vi "test_libssh2_session_blocking.vi"() -> ()   [LabVIEW 2013, in "libssh2_tests.lvlib"]
uses:
  libssh2/libssh2_init_default.vi
  libssh2_tests.lvlib
  <vilib>/addons/_JKI Toolkits/Caraya/classes/Test/Test.lvclass
  libssh2/libssh2.lvlib
  <vilib>/addons/_JKI Toolkits/Caraya/classes/Assert/Assert.lvclass
panel:
  out "error out":errorcluster
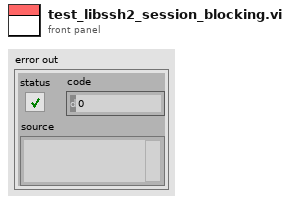
[diagram p1: front panel]
types:
  T1 = typedef "libssh2.lvlib/Session Refnum.ctl" = refnum<k1>
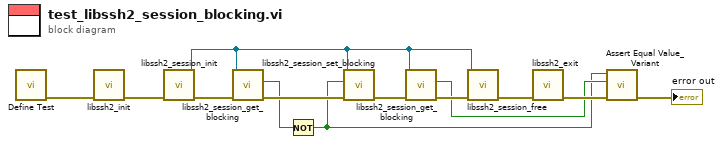
[diagram p0: block diagram]
diagram:
  n1 = call <vilib>:"Define Test.vi"() -> ("error out"=w8:errorcluster)  [unwired: 10 in, 1 out]
  n2 = call-poly "libssh2_init.vi"("error in (no error)"=w8) -> ("error out"=w12:errorcluster)  [unwired: 10 in]
  n3 = call "libssh2_session_init.vi"("error in (no error)"=w12) -> ("error out"=w5:errorcluster, "session"=w4:T1)  [unwired: 9 in]
  n4 = call "libssh2_session_get_blocking.vi"("error in (no error)"=w5, "session"=w4) -> ("error out"=w6:errorcluster, "blocking"=w3:bool)  [unwired: 8 in]
  n5 = Not(x=w3) -> (.not. x?=w1:bool)
  n6 = call "libssh2_session_set_blocking.vi"("error in (no error)"=w6, "blocking"=w1, "session"=w4) -> ("error out"=w10:errorcluster)  [unwired: 8 in]
  n7 = call "libssh2_session_get_blocking.vi"("error in (no error)"=w10, "session"=w4) -> ("error out"=w7:errorcluster, "blocking"=w2:bool)  [unwired: 8 in]
  n8 = call "libssh2_session_free.vi"("error in (no error)"=w7, "session"=w4) -> ("error out"=w11:errorcluster)  [unwired: 9 in]
  n9 = call "libssh2_exit.vi"("error in (no error)"=w11) -> ("error out"=w9:errorcluster)  [unwired: 10 in]
  n10 = call <vilib>:"Assert Equal Value_Variant.vi"("error in (no error)"=w9, "Y"=w2, "X"=w1) -> ("error out"=→"error out":errorcluster)  [unwired: 7 in, 1 out]
